vi "plot_ai.vi"() -> ()   [LabVIEW 2009]
uses:
  <vilib>/DAQmx/create/channels.llb/DAQmx Create Channel (AI-Voltage-Basic).vi
  <vilib>/DAQmx/read.llb/DAQmx Read (Analog DBL 1Chan 1Samp).vi
panel:
  out "Waveform Chart":dbl(graph)
  in  "stop":bool
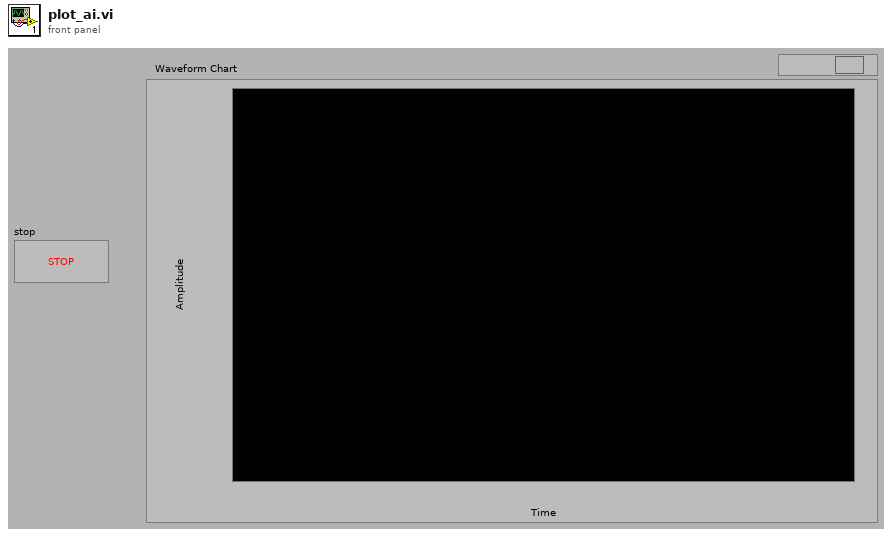
[diagram p1: front panel]
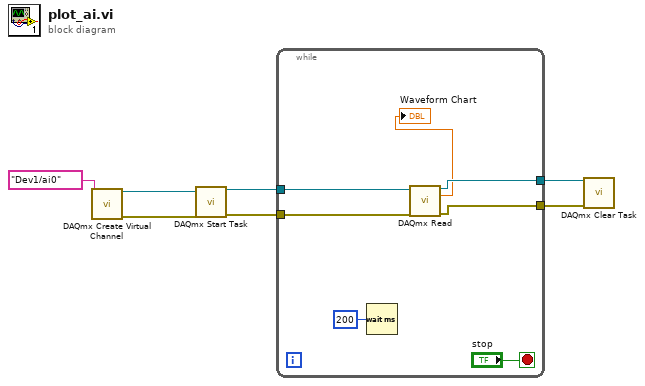
[diagram p0: block diagram]
diagram:
  n1 = call-poly <vilib>:"DAQmx Create Virtual Channel.vi"("physical channels"=tag "Dev1/ai0") -> ("task out"=w7:refnum<k21>, "error out"=w6:errorcluster)  [unwired: 13 in]
  n2 = call <vilib>:"DAQmx Start Task.vi"("task/channels in"=w7, "error in"=w6) -> ("task out"=w5:refnum<k21>, "error out"=w4:errorcluster)  [unwired: 12 in]
  n3 = while {
    tunnel: w5 -> [w14]
    tunnel: w4 -> [w13]
    tunnel: [w12] -> w3
    tunnel: [w11] -> w2
    stop <- "stop" stop-if-true
    n4 = Wait (ms)(milliseconds to wait=u32 200) -> ()  [unwired: 1 out]
    n5 = call-poly <vilib>:"DAQmx Read.vi"("task/channels in"=w14, "error in"=w13) -> ("task out"=w11:refnum<k21>, "data"=→"Waveform Chart":dbl, "error out"=w12:errorcluster)  [unwired: 11 in]
  }
  n6 = call <vilib>:"DAQmx Clear Task.vi"("task in"=w2, "error in"=w3) -> ()  [unwired: 13 in, 1 out]
